vi "WaitAny Helper Async.vi"(9 "Timeout":i32, 10 "Forwarded Event":refnum<user-event>, 11 "Event Reg":refnum<event-registration>) -> ()   [LabVIEW 2020, in "Promises.lvlib" / "Future.lvclass"]
uses:
  Future.lvclass
  Result.ctl
  Result State.ctl
  Promises.lvlib
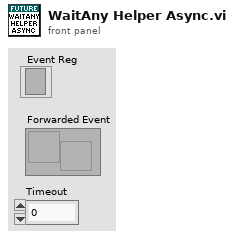
[diagram p1: front panel]
types:
  T1 = typedef "Promises.lvlib/Result.ctl" = cluster{"State":T2, "Value":refnum<class>}
  T2 = typedef "Promises.lvlib/Result State.ctl" = enum16{"Unset", "Error", "Success"}
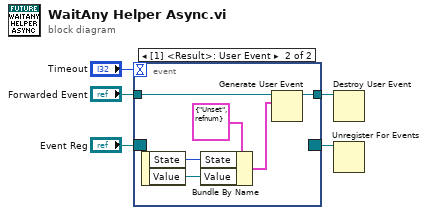
[diagram p0: block diagram]
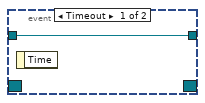
[diagram p2: hidden frame]
diagram:
  n1 = event shown="[1] <Result>: User Event" {
    selector: "Event Reg" -> [_ _]
    dyn-events: [_ _] -> w2
    timeout: "Timeout" -> [_ _]
    tunnel: "Forwarded Event" -> [w6 w12]
    tunnel: [w6 w7] -> w1
    event Timeout {
      n2 = event-data() -> ()  [unwired: 1 in, 1 out]
    }
    event User Event {
      n3 = event-data() -> ("State"=w9:T2, "Value"=w8:refnum<class>)  [unwired: 1 in]
      n4 = Bundle By Name(cluster=T1 {"State"=enum."Unset", "Value"=refnum} ("event data"), "State"=w9, "Value"=w8) -> (w10:T1)
      n5 = Generate User Event(user event=w12, event data cluster=w10) -> (user event out=w7:refnum<user-event>)  [unwired: 2 in, 1 out]
    }
  }
  n6 = Destroy User Event(user event=w1) -> ()  [unwired: 1 in, 1 out]
  n7 = Unregister For Events(event registration refnum=w2) -> ()  [unwired: 1 in, 1 out]
